vi "AutoCAD cmds 64bit.vi"(6 "AutoCAD cmd":T3, 8 "error in (no error)":errorcluster, 9 "Command":string, 10 "Mathcad Output":T2, 11 "DesignRequest":T1) -> (0 "error out":errorcluster, 2 "IsQuiescent":bool, 3 "DesignRequest out":T1)   [LabVIEW 2015]
uses:
  AutoCAD cmds.ctl
  Design Request.ctl
  Variable cluster.ctl
  AguaClara Library.lvlib
panel:
  out "new doc error":errorcluster
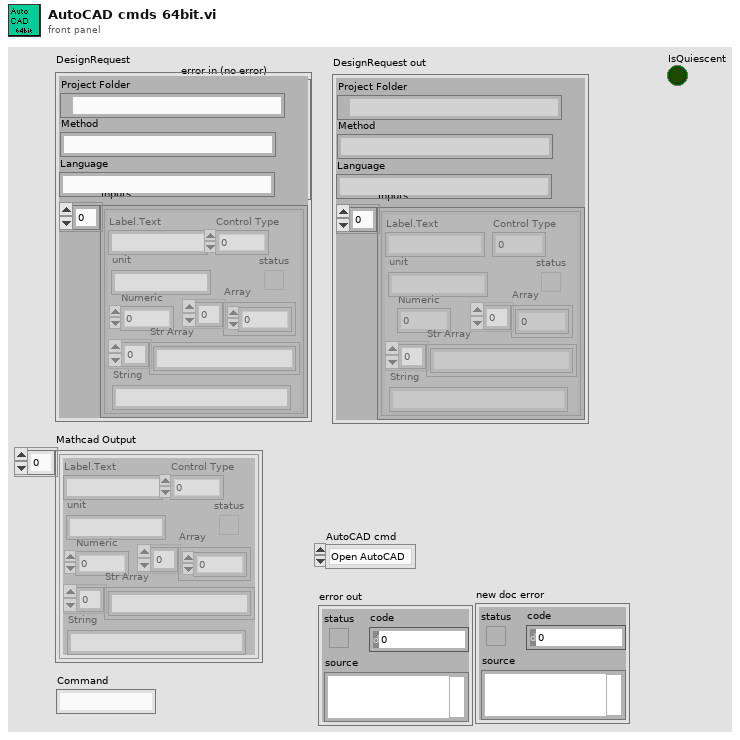
[diagram p1: front panel]
types:
  T1 = typedef "Design Request.ctl" = cluster{"Project Folder":path, "Method":string, "Inputs":T2, "Language":string}
  T2 = typedef "Variable cluster.ctl" = cluster{"Label.Text":string, "Control Type":u32, "Numeric":dbl, "Array":dbl[], "status":bool, "Str Array":string[], "String":string, "unit":string}[]
  T3 = typedef "AguaClara Library.lvlib/AutoCAD cmds.ctl" = enum16{"Open AutoCAD", "New Document", "Send Command", "Send Command Array", "Close Doc", "Quit"}
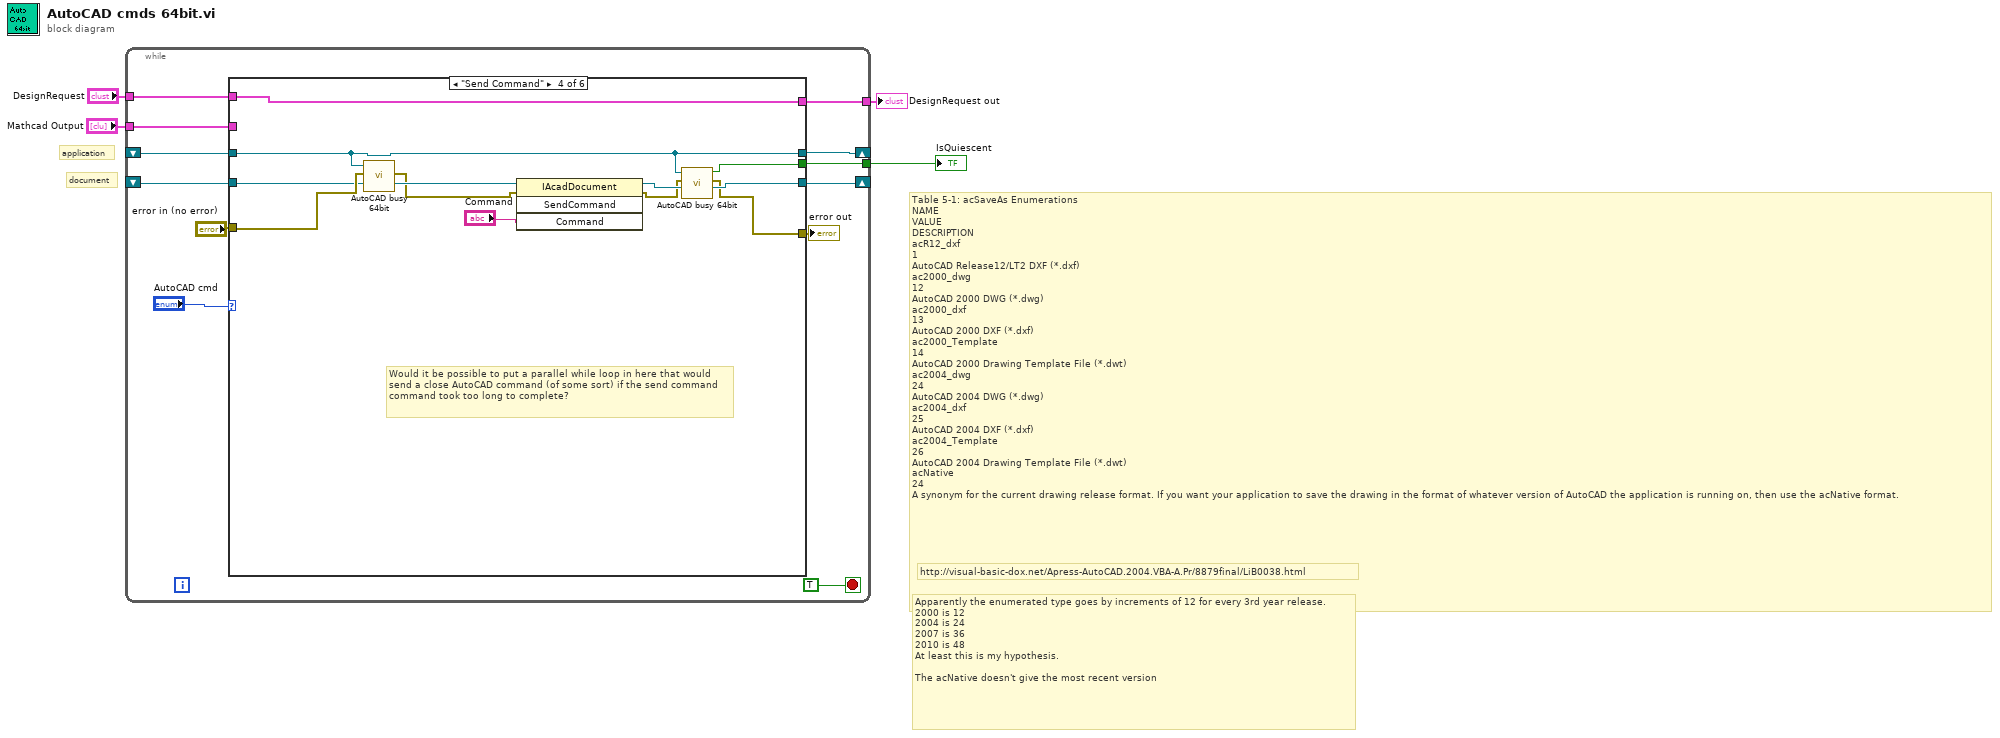
[diagram p0: block diagram]
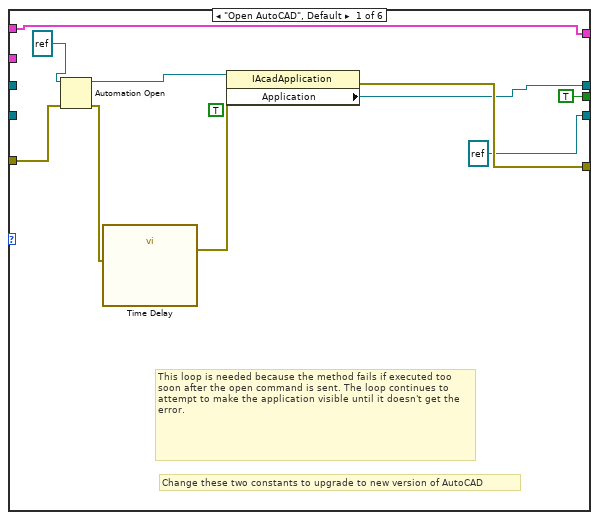
[diagram p2: hidden frame]
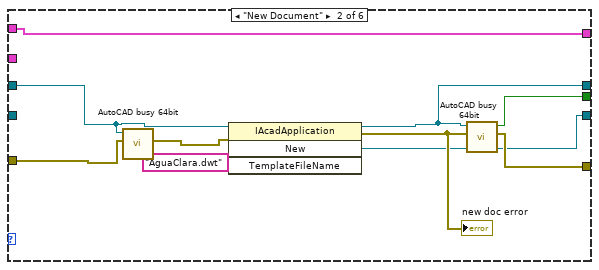
[diagram p3: hidden frame]
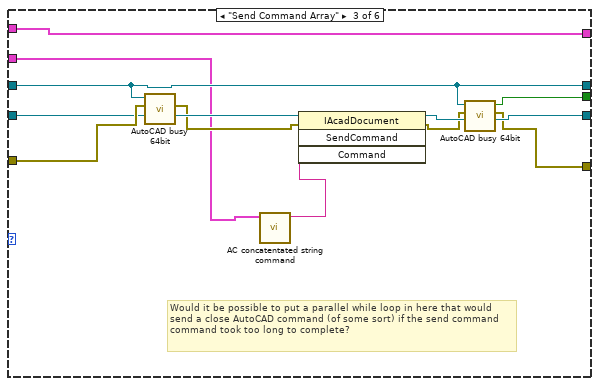
[diagram p4: hidden frame]
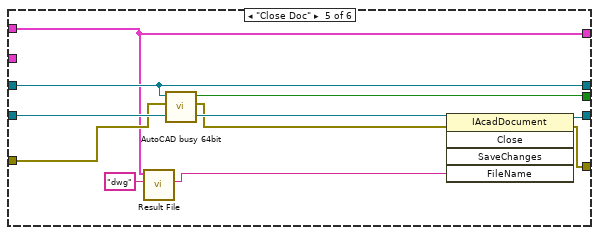
[diagram p5: hidden frame]
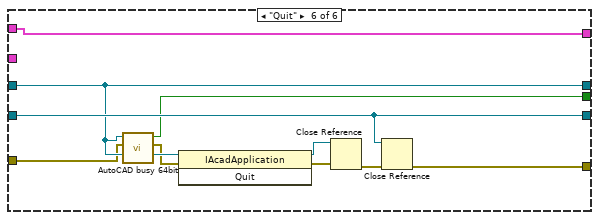
[diagram p6: hidden frame]
diagram:
  # "Apparently the enumerated type goes by increments of 12 for every 3rd year release.\n2000 is 12\n2004 is 24\n2007 is 36\n2010 is 48\nAt least this is my hypothesis. \n\nThe acNative doesn't give the most recent version"
  # "http://visual-basic-dox.net/Apress-AutoCAD.2004.VBA-A.Pr/8879final/LiB0038.html"
  # "Table 5-1: acSaveAs Enumerations\nNAME\nVALUE\nDESCRIPTION\nacR12_dxf\n1\nAutoCAD Release12/LT2 DXF (*.dxf)\nac2000_dwg\n12\nAutoCAD 2000 DWG (*.dwg)\nac2000_dxf\n13\nAutoCAD 2000 DXF (*.dxf)\nac2000_Template\n14\nAutoCAD 2000 Drawing Template File (*.dwt)\nac2004_dwg\n24\nAutoCAD 2004 DWG (*.dwg)\nac2004_dxf\n25\nAutoCAD 2004 DXF (*.dxf)\nac2004_Template\n26\nAutoCAD 2004 Drawing Template File (*.dwt)\nacNative\n24\nA synonym for the current drawing release format. If you want your application to save the drawing in the format of whatever version of AutoCAD the application is running on, then use the acNative format."
  # "document"
  # "application"
  n1 = while {
    shift-right: [w15] -> _
    shift-left: _ -> [w10]
    shift-right: [w12] -> _
    shift-left: _ -> [w11]
    tunnel: [w8] -> w4
    tunnel: [w7] -> w3
    tunnel: "DesignRequest" -> [w6]
    tunnel: "Mathcad Output" -> [w5]
    stop <- TRUE stop-if-true
    n2 = case shown="\"Send Command\"" "AutoCAD cmd" {
      tunnel: [w23 w32 w42 w53 w64 w72] -> w15
      tunnel: "error in (no error)" -> [w20 w34 w47 w57 w63 w71]
      tunnel: [w26 w36 w40 w51 w65 w73] -> w13
      tunnel: [refnum<k7> refnum ("Add") w29 w44 w54 w66 w74] -> w12
      tunnel: w11 -> [_ _ w46 w56 w67 w74]
      tunnel: w10 -> [_ w33 w42 w53 w64 w72]
      tunnel: [TRUE ("IsQuiescent") w35 w39 w50 w61 w69] -> w8
      tunnel: [w17 w27 w37 w49 w58 w68] -> w7
      tunnel: w6 -> [w17 w27 w37 w49 w58 w68]
      tunnel: w5 -> [_ _ w38 _ _ _]
      frame "Open AutoCAD", Default {
        (unwired) TRUE ("Visible")
        # "This loop is needed because the method fails if executed too soon after the open command is sent. The loop continues to attempt to make the application visible until it doesn't get the error."
        # "Change these two constants to upgrade to new version of AutoCAD"
        n3 = Automation Open(error in (no error)=w20, Automation Refnum=refnum<k7> refnum ("reference")) -> (Automation Refnum=w21:refnum<k7>, error out=w19:errorcluster)  [unwired: 2 in]
        n4 = call "Time Delay"("error in (no error)"=w19) -> ("error out"=w18:errorcluster)  [unwired: 10 in]
        n5 = property class="IAcadApplication"(reference=w21, error in=w18) -> (error out=w26:errorcluster, "Application"=w23:refnum<k7>)  [unwired: 1 out]
      }
      frame "New Document" {
        n6 = call "AutoCAD busy 64bit.vi"("error in (no error)"=w34, "Application"=w33) -> ("error out"=w31:errorcluster)  [unwired: 4 in, 1 out]
        n7 = invoke class="IAcadApplication" method="New"(reference=w33, error in=w31, "TemplateFileName"="AguaClara.dwt") -> (reference out=w32:refnum<k7>, error out=w30:errorcluster, "New"=w29:refnum<k7>)  [unwired: 1 in, 1 out]
        "new doc error" <- w30
        n8 = call "AutoCAD busy 64bit.vi"("error in (no error)"=w30, "Application"=w32) -> ("error out"=w36:errorcluster, "IsQuiescent"=w35:bool)  [unwired: 4 in]
      }
      frame "Send Command Array" {
        # "Would it be possible to put a parallel while loop in here that would send a close AutoCAD command (of some sort) if the send command command took too long to complete?"
        n9 = call "AutoCAD busy 64bit.vi"("error in (no error)"=w47, "Application"=w42) -> ("error out"=w45:errorcluster)  [unwired: 4 in, 1 out]
        n10 = call "AC concatentated string command.vi"("MathCAD results"=w38) -> ("AC concatenated string"=w43:string)  [unwired: 10 in]
        n11 = invoke class="IAcadDocument" method="SendCommand"(reference=w46, error in=w45, "Command"=w43) -> (reference out=w44:refnum<k7>, error out=w41:errorcluster)  [unwired: 1 in, 2 out]
        n12 = call "AutoCAD busy 64bit.vi"("error in (no error)"=w41, "Application"=w42) -> ("error out"=w40:errorcluster, "IsQuiescent"=w39:bool)  [unwired: 4 in]
      }
      frame "Send Command" {
        # "Would it be possible to put a parallel while loop in here that would send a close AutoCAD command (of some sort) if the send command command took too long to complete?"
        n13 = call "AutoCAD busy 64bit.vi"("error in (no error)"=w57, "Application"=w53) -> ("error out"=w55:errorcluster)  [unwired: 4 in, 1 out]
        n14 = invoke class="IAcadDocument" method="SendCommand"(reference=w56, error in=w55, "Command"="Command") -> (reference out=w54:refnum<k7>, error out=w52:errorcluster)  [unwired: 1 in, 2 out]
        n15 = call "AutoCAD busy 64bit.vi"("error in (no error)"=w52, "Application"=w53) -> ("error out"=w51:errorcluster, "IsQuiescent"=w50:bool)  [unwired: 4 in]
      }
      frame "Close Doc" {
        n16 = call "Result File.vi"("File Type"="dwg", "DesignRequest"=w58) -> ("File string"=w59:string)  [unwired: 8 in, 1 out]
        n17 = call "AutoCAD busy 64bit.vi"("error in (no error)"=w63, "Application"=w64) -> ("error out"=w62:errorcluster, "IsQuiescent"=w61:bool)  [unwired: 4 in]
        n18 = invoke class="IAcadDocument" method="Close"(reference=w67, error in=w62, "FileName"=w59) -> (reference out=w66:refnum<k7>, error out=w65:errorcluster)  [unwired: 2 in, 3 out]
      }
      frame "Quit" {
        n19 = call "AutoCAD busy 64bit.vi"("error in (no error)"=w71, "Application"=w72) -> ("error out"=w70:errorcluster, "IsQuiescent"=w69:bool)  [unwired: 4 in]
        n20 = invoke class="IAcadApplication" method="Quit"(reference=w72, error in=w70) -> (reference out=w77:refnum<k7>, error out=w76:errorcluster)  [unwired: 1 in, 1 out]
        n21 = Close Reference(reference=w77, error in (no error)=w76) -> (error out=w75:errorcluster)
        n22 = Close Reference(reference=w74, error in (no error)=w75) -> (error out=w73:errorcluster)
      }
    }
    "error out" <- w13
  }
  "IsQuiescent" <- w4
  "DesignRequest out" <- w3
